vi "Create Controls in Configuration.vi"(8 "error in (no error)":errorcluster, 9 "VI Refnum":refnum<vi>, 10 "Ctl Refnum":refnum<vi>, 11 "Cluster Ref":refnum<vi>) -> (0 "error out":errorcluster, 3 "Control out":refnum<vi>)   [LabVIEW 2021, in "Migrator.lvlib"]
uses:
  Migrator.lvlib
  <vilib>/Utility/miscctls.llb/LVPositionTypeDef.ctl
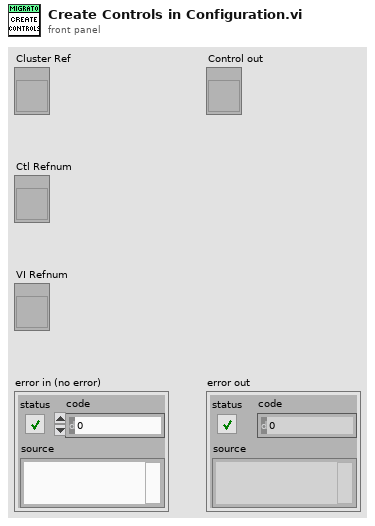
[diagram p1: front panel]
types:
  T1 = typedef "LVPositionTypeDef.ctl" = cluster{"Left":i32, "Top":i32}
  T2 = enum32{"not a typedef", "typedef", "strict typedef", "class private data"}
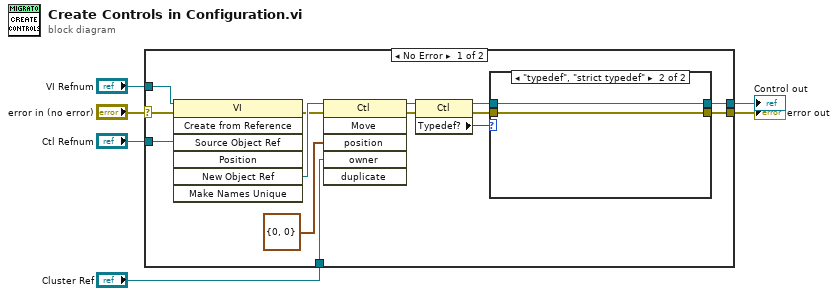
[diagram p0: block diagram]
diagram:
  n1 = case shown="No Error" "error in (no error)" {
    selector: "error in (no error)" -> [w13 w25]
    tunnel: [w18 _] -> w6
    tunnel: [w17 w25] -> w5
    tunnel: "Ctl Refnum" -> [w16 _]
    tunnel: "Cluster Ref" -> [w15 _]
    tunnel: "VI Refnum" -> [w14 _]
    frame No Error {
      n2 = invoke class="VI" method="Create from Reference"(reference=w14, error in=w13, "Source Object Ref"=w16) -> (error out=w10:errorcluster, "New Object Ref"=w11:refnum<vi>)  [unwired: 4 in, 5 out]
      n3 = invoke class="Ctl" method="Move"(reference=w11, error in=w10, "position"=T1 {"Left"=0, "Top"=0}, "owner"=w15) -> (reference out=w19:refnum<vi>, error out=w7:errorcluster)  [unwired: 2 in, 4 out]
      n4 = property class="Ctl"(reference=w19, error in=w7) -> (reference out=w8:refnum<vi>, error out=w9:errorcluster, "Typedef?"=w20:T2)
      n5 = case shown="\"typedef\", \"strict typedef\"" w20 {
        tunnel: w9 -> [w22 w23]
        tunnel: [w22 w23] -> w17
        tunnel: [w21 w24] -> w18
        tunnel: w8 -> [w21 w24]
        frame "not a typedef", Default {
        }
        frame "typedef", "strict typedef" {
        }
      }
    }
    frame Error {
    }
  }
  "Control out" <- w6
  "error out" <- w5
